vi "GoTo Field (PID).vi"() -> ()   [LabVIEW 2009, in "Varian Magnet.lvclass"]
uses:
  Varian Magnet.lvclass
  Varian Magnet.lvclass/Varian Magnet.ctl
  Varian/Varian.lvlib
panel:
  in  "D":dbl
  in  "I":dbl
  in  "P":dbl=8.0
  out "Varian Magnet out":refnum<class "Varian Magnet.lvclass">
  out "error out":errorcluster
  out "Waveform Chart":dbl[unit](graph)
  out "Current Field":dbl[unit]
  in  "Desired Field":dbl
  in  "stop":bool
  in  "error in (no error)":errorcluster
  in  "Varian Magnet.lvclass In":refnum<class "Varian Magnet.lvclass">
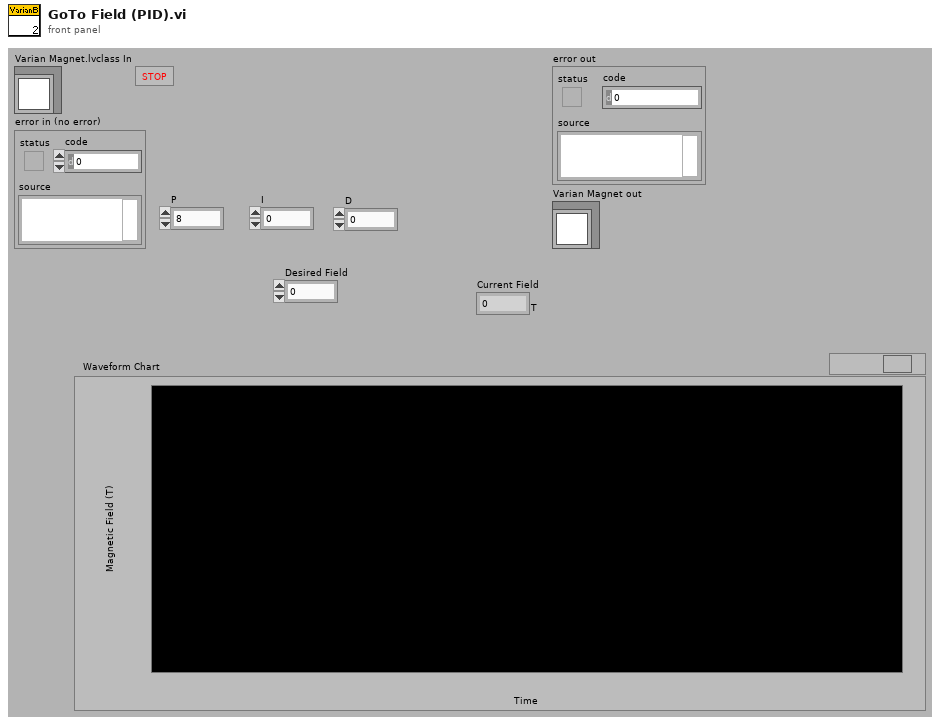
[diagram p1: front panel]
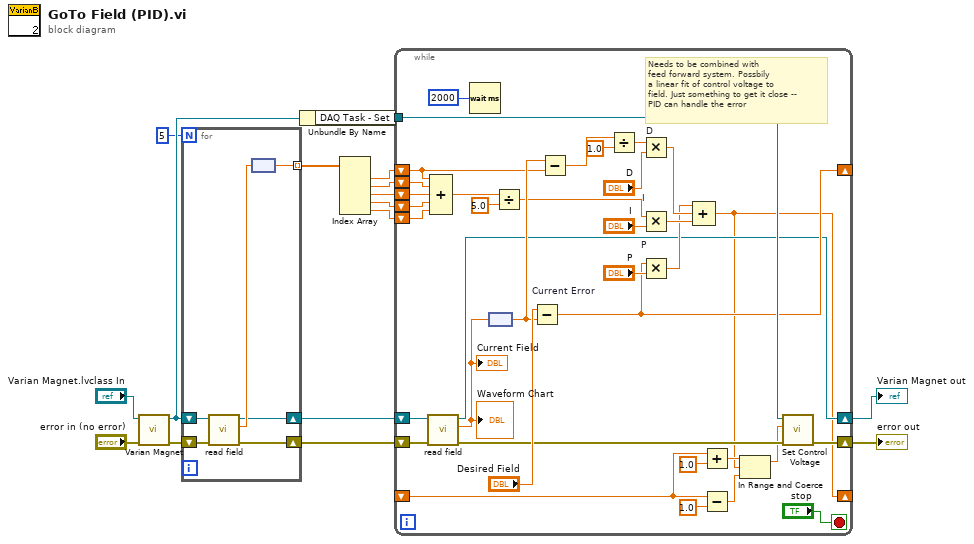
[diagram p0: block diagram]
diagram:
  n1 = call "Varian Magnet.vi"("error in (no error)"="error in (no error)", "Varian Magnet in"="Varian Magnet.lvclass In") -> ("error out"=w13:errorcluster, "Varian Magnet out"=w12:refnum<class "Varian Magnet.lvclass">)  [unwired: 8 in]
  n2 = for {
    N: 5 -> [_]
    shift-right: [w18] -> w7
    shift-left: w12 -> [w22]
    shift-right: [w20] -> w11
    shift-left: w13 -> [w21]
    tunnel: [w17] -> w1 mode=indexing
    n3 = call "read field.vi"("error in (no error)"=w21, "Varian Magnet.lvclass In"=w22) -> ("error out"=w20:errorcluster, "Field"=w19:dbl[unit], "Varian Magnet.lvclass Out"=w18:refnum<class "Varian Magnet.lvclass">)  [unwired: 7 in]
    n4 = node(w19) -> (w17:dbl)
  }
  n5 = Unbundle By Name(w12) -> ("DAQ Task - Set"=w14:refnum<k21>)
  n6 = Index Array(array=w1) -> (element #1=w6:dbl, element #2=w5:dbl, element #3=w4:dbl, element #4=w3:dbl, element #5=w2:dbl)  [unwired: 5 in]
  n7 = while {
    shift-right: [w32] -> w9
    shift-left: w7 -> [w56]
    shift-right: [w33] -> w10
    shift-left: w11 -> [w57]
    shift-right: [w34] -> _
    shift-left: w6 -> [w47]
    shift-left: w5 -> [w54]
    shift-left: w4 -> [w53]
    shift-left: w3 -> [w52]
    shift-left: w2 -> [w51]
    tunnel: w14 -> [w35]
    shift-right: [w23] -> _
    shift-left: _ -> [w27]
    stop <- "stop" stop-if-true
    # "Needs to be combined with \nfeed forward system. Possbily\na linear fit of control voltage to\nfield. Just something to get it close --\nPID can handle the error"
    n8 = call "read field.vi"("error in (no error)"=w57, "Varian Magnet.lvclass In"=w56) -> ("error out"=w36:errorcluster, "Field"=w31:dbl[unit], "Varian Magnet.lvclass Out"=w32:refnum<class "Varian Magnet.lvclass">)  [unwired: 7 in]
    "Current Field" <- w31
    "Waveform Chart" <- w31
    n9 = Compound Arithmetic op=ADD(w47, w54, w53, w52, w51) -> (w50:dbl)
    n10 = Wait (ms)(milliseconds to wait=u32 2000) -> ()  [unwired: 1 out]
    n11 = node(w31) -> (w48:dbl)
    n12 = Divide(x=w50, y=5.0) -> (x/y=w44:dbl)
    n13 = Subtract "Current Error"(x="Desired Field", y=w48) -> (x-y=w34:dbl)
    n14 = Subtract(x=w48, y=w47) -> (x-y=w46:dbl)
    n15 = Divide(x=w46, y=1.0) -> (x/y=w43:dbl)
    n16 = Multiply "D"(x=w43, y="D") -> (x*y=w38:dbl)
    n17 = Multiply "I"(x=w44, y="I") -> (x*y=w39:dbl)
    n18 = Multiply "P"(x=w34, y="P") -> (x*y=w37:dbl)
    n19 = Compound Arithmetic op=ADD(w37, w38, w39) -> (w23:dbl)
    n20 = Add(x=w27, y=1.0) -> (x+y=w29:dbl)
    n21 = Subtract(x=w27, y=1.0) -> (x-y=w28:dbl)
    n22 = In Range and Coerce(upper limit=w29, x=w23, lower limit=w28) -> (coerced(x)=w24:dbl)  [unwired: 1 out]
    n23 = call "Set Control Voltage.vi"("error in"=w36, "Control Voltage"=w24, "task in"=w35) -> ("error out"=w33:errorcluster)  [unwired: 8 out]
  }
  "error out" <- w10
  "Varian Magnet out" <- w9
